vi "Vision Processing.vi"(2 "error in (no error)":errorcluster, 3 "Camera Type":enum16{"206", "1011"}(ring)=enum."1011", 4 "Camera Name":string="Camera") -> (0 "Target Info":T1(array[cluster]))   [LabVIEW 2012]
uses:
  Robot Global Data.vi
  <vilib>/vision/NI_Vision_Development_Module.lvlib
panel:
  in  "View Zoom":bool
  in  "Make Target Info":T1(array[cluster])
  in  "Don't use camera?":bool=TRUE
  out "zoomed binary":T2(plugin-control)
  in  "View":bool
  in  "Area Size Limit":i32=444
  in  "Particle Count Limit":i32=8
  in  "Score Limits":T3={"Rect Coverage"=76.0, "Aspect Ratio"=70.0, "X Edge Strength"=60.0, "Y Edge Strength"=40.0}
  in  "Processing":enum32{"Color", "Intensity", "Intensity Open"}(tab)
  in  "Luminance":i32=200
  in  "Saturation":i32=50
  in  "Hue":i32(knob)=121 scale=0.0..255.0
  in  "Margins":cluster{"Hue":i32, "Sat":i32, "Lum":i32}={"Hue"=40, "Sat"=40, "Lum"=20} {"Sat" scale=0.0..40.0; "Lum" scale=0.0..40.0; "Hue" scale=0.0..40.0}
  in  "Range":cluster{"Lower value":sgl, "Upper value":sgl}={"Lower value"=150.0, "Upper value"=255.0} {"Lower value" scale=0.0..255.0; "Upper value" scale=0.0..255.0}
  in  "Range":cluster{"Lower value":sgl, "Upper value":sgl}={"Lower value"=150.0, "Upper value"=255.0} {"Lower value" scale=0.0..255.0; "Upper value" scale=0.0..255.0}
  in  "View":bool
  out "Processed Image":T2(plugin-control)
  out "Original Image":T2(plugin-control)
  # "Instructions:\nProcessing the reflective tape that is illuminated by a ring light can be based\non color or light intensity.\nParticles within the image are scored by rectangle coverage, aspect ratio, and\nfor being hollow with a bold edge. A particle is considered a target if all scores\nare above the score limits. Particles can be annotated -- surrounded by\na rectangle and scores drawn to the left .\nTo control the number of particles being scored, use the count limit and the size\nlimit."
  # "To debug, Enable using the View button.\nFor color processing, you can click in the image to select the color for processing."
  # "Enable by clicking the View button.\nGreen scores are above the limit, orange are below. Inner/outer rect\nindicates all passed."
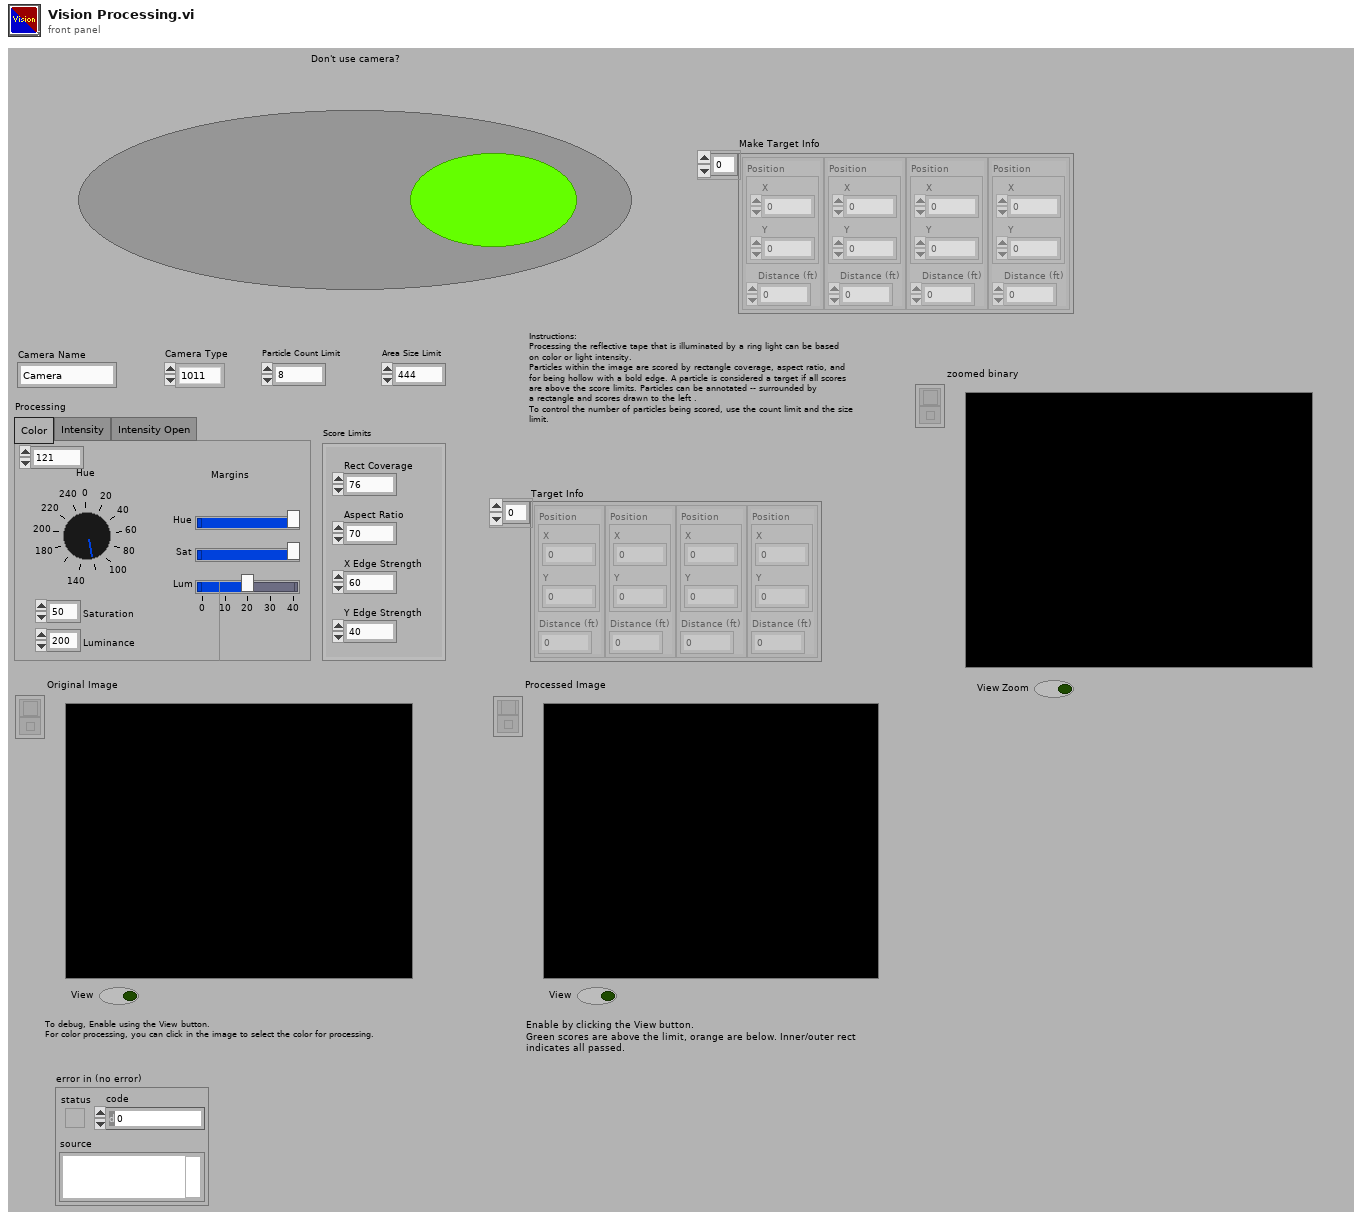
[diagram p1: front panel]
types:
  T1 = cluster{"Position":cluster{"X":dbl, "Y":dbl}, "Distance (ft)":dbl}[]
  T2 = typedef "IMAQ Image.ctl" = refnum<image>
  T3 = cluster{"Rect Coverage":dbl, "Aspect Ratio":dbl, "X Edge Strength":dbl, "Y Edge Strength":dbl}
  T4 = enum32{"AutoM", "Close", "Dilate", "Erode", "Gradient", "Gradient out", "Gradient in", "Hit miss", "Open", "PClose", "POpen", "Thick", "Thin"}
  T5 = typedef "Image Type" = u32
  T6 = typedef "WPI_CameraDevRef.ctl" = cluster{"Camera Address":string, "CameraStatus":errorcluster, "Acquire Image Notifier":refnum<notifier>}
  T7 = typedef "WPI_CameraImageSize.ctl" = enum16{"640x480", "320x240", "160x120"}
  T8 = cluster{cluster{"Left":dbl, "Top":dbl, "Right":dbl, "Bottom":dbl}, dbl[]}[]
  T9 = cluster{"Left":dbl, "Top":dbl, "Right":dbl, "Bottom":dbl}
  T10 = cluster{"Target Center (-1 to 1)":cluster{"X":dbl, "Y":dbl}, "Distance (ft)":dbl}
  T11 = cluster{"Target Center (-1 to 1)":cluster{"X":dbl, "Y":dbl}, "Distance (ft)":dbl}[]
  T12 = cluster{"Scored Particle Info[0]":cluster{cluster{"Left":dbl, "Top":dbl, "Right":dbl, "Bottom":dbl}, dbl[]}, "Scored Particle Info[1]":cluster{cluster{"Left":dbl, "Top":dbl, "Right":dbl, "Bottom":dbl}, dbl[]}, "Scored Particle Info[2]":cluster{cluster{"Left":dbl, "Top":dbl, "Right":dbl, "Bottom":dbl}, dbl[]}, "Scored Particle Info[3]":cluster{cluster{"Left":dbl, "Top":dbl, "Right":dbl, "Bottom":dbl}, dbl[]}, "Scored Particle Info[4]":cluster{cluster{"Left":dbl, "Top":dbl, "Right":dbl, "Bottom":dbl}, dbl[]}, "Scored Particle Info[5]":cluster{cluster{"Left":dbl, "Top":dbl, "Right":dbl, "Bottom":dbl}, dbl[]}, "Scored Particle Info[6]":cluster{cluster{"Left":dbl, "Top":dbl, "Right":dbl, "Bottom":dbl}, dbl[]}, "Scored Particle Info[7]":cluster{cluster{"Left":dbl, "Top":dbl, "Right":dbl, "Bottom":dbl}, dbl[]}, "Scored Particle Info[8]":cluster{cluster{"Left":dbl, "Top":dbl, "Right":dbl, "Bottom":dbl}, dbl[]}}
  T13 = cluster{cluster{"Left":dbl, "Top":dbl, "Right":dbl, "Bottom":dbl}, dbl[]}
  T14 = cluster{"Position":cluster{"X":dbl, "Y":dbl}, "Distance (ft)":dbl}
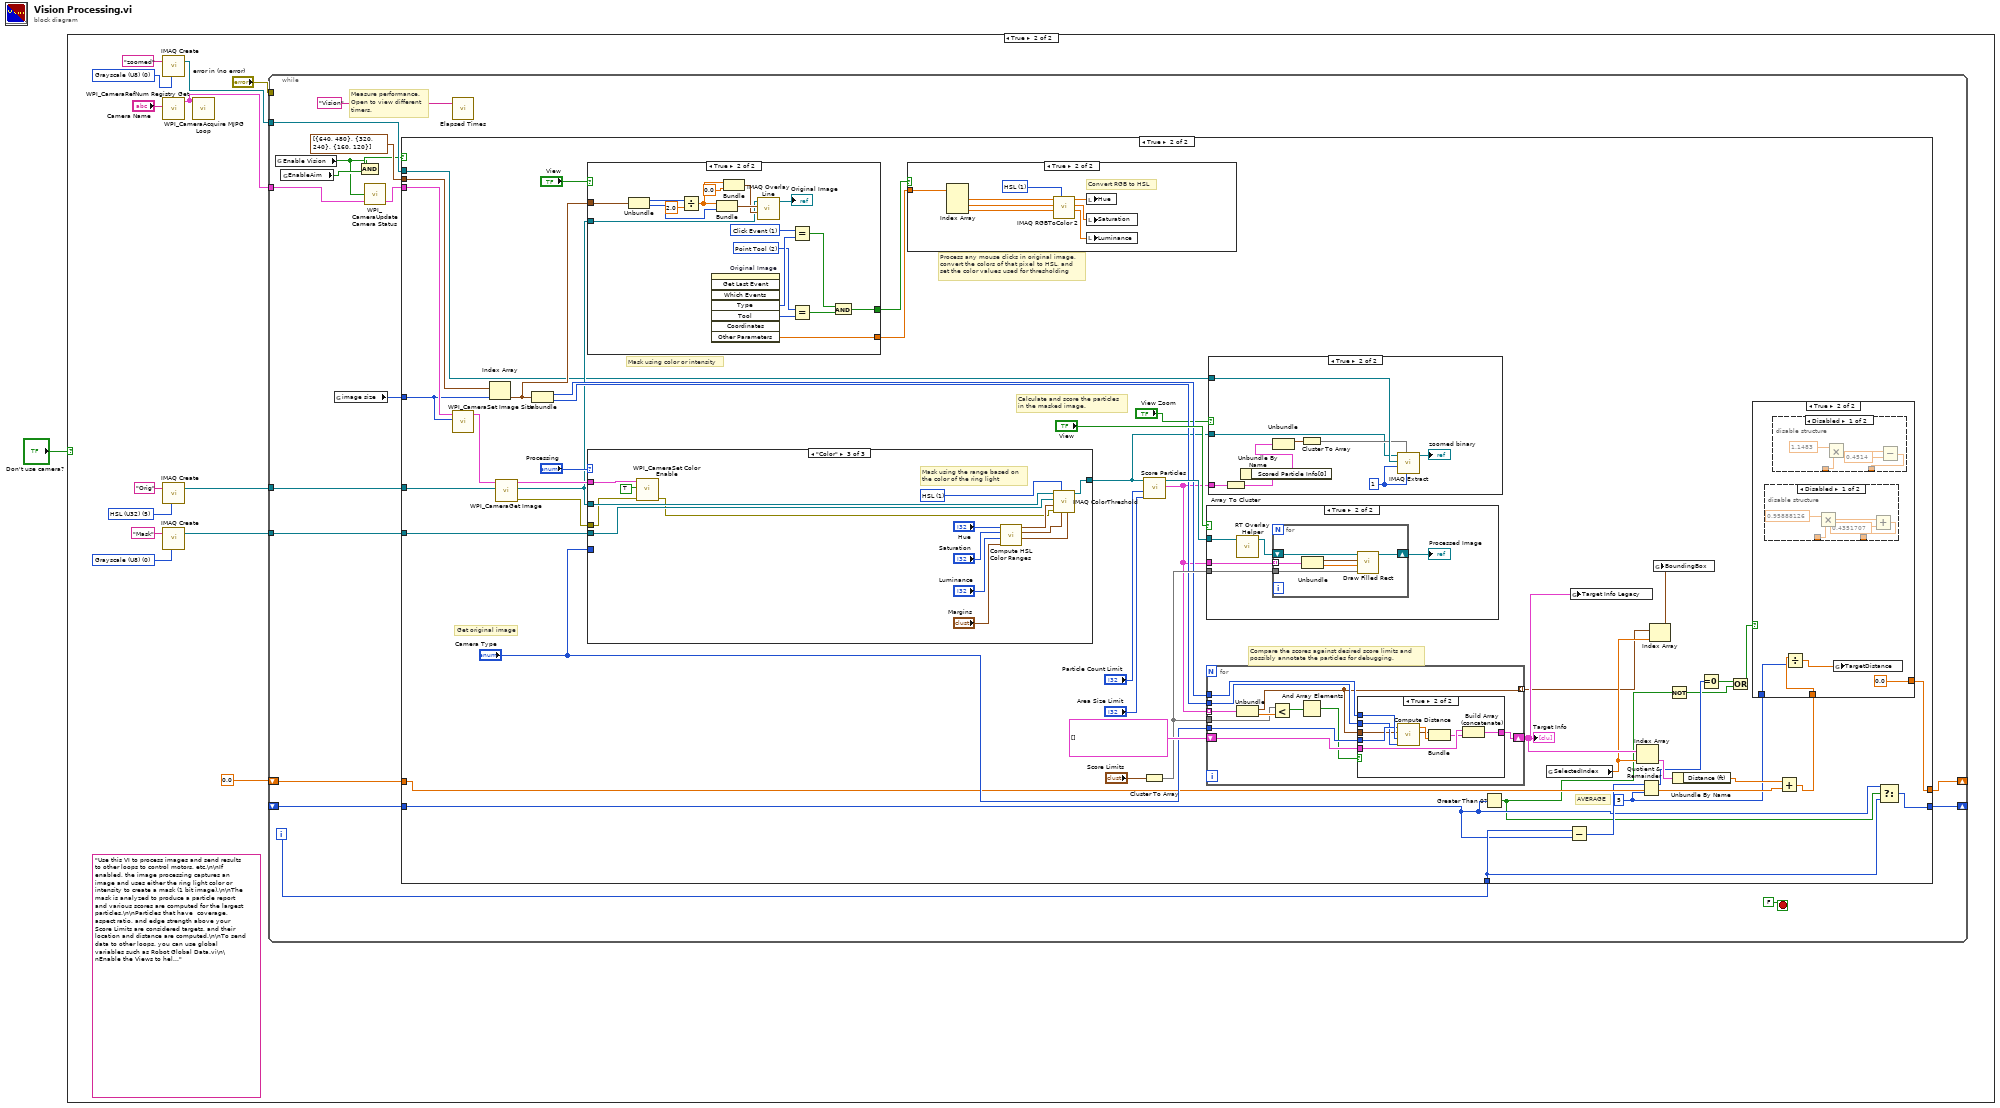
[diagram p0: block diagram]
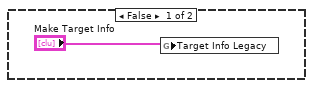
[diagram p2: hidden frame]
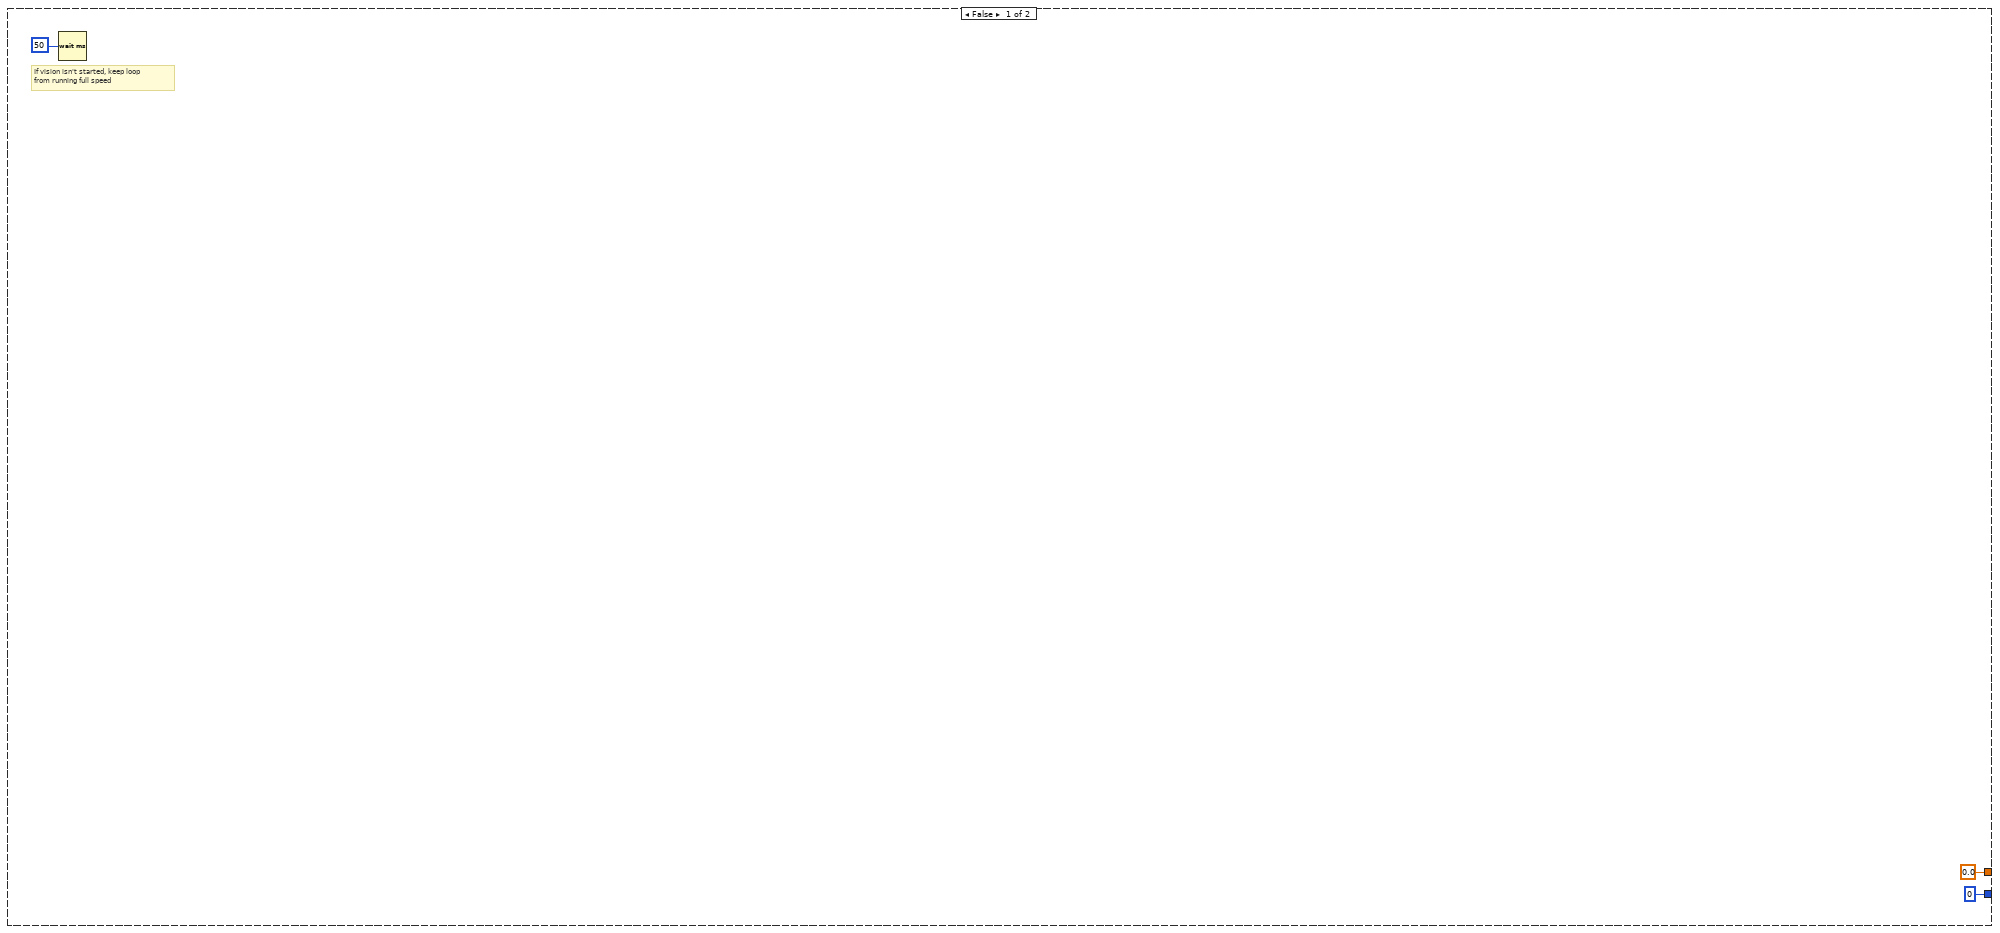
[diagram p3: hidden frame]
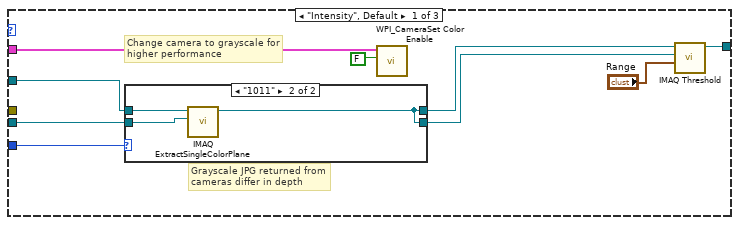
[diagram p9: hidden frame]
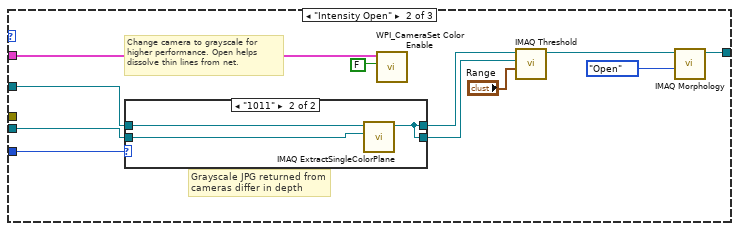
[diagram p11: hidden frame]
diagram:
  n1 = case shown="True" "Don't use camera?" {
    frame False {
      n2 = global write "Robot Global Data.vi" "Target Info Legacy"("Make Target Info") -> ()
    }
    frame True {
      w5 = T5 0 items=["Grayscale (U8)", "Grayscale (I16)", "Grayscale (SGL)", "Complex (CSG)", "RGB (U32)", "HSL (U32)", "RGB (U64)", "Grayscale (U16)"] ("Image Type")
      w9 = T5 0 items=["Grayscale (U8)", "Grayscale (I16)", "Grayscale (SGL)", "Complex (CSG)", "RGB (U32)", "HSL (U32)", "RGB (U64)", "Grayscale (U16)"] ("Image Type")
      (unwired) "Use this VI to process images and send results to other loops to control motors, etc.\n\nIf enabled, the image processing captures an image and uses either the ring light color or intensity to create a mask (1 bit image).\n\nThe mask is analyzed to produce a particle report and various scores are computed for the largest particles.\n\nParticles that have  coverage, aspect ratio, and edge strength above your Score Limits are considered targets, and their location and distance are computed.\n\nTo send data to other loops, you can use global variables such as Robot Global Data.vi\n\nEnable the Views to help debug color settings. Disable the View to speed up processing."
      w14 = T5 5 items=["Grayscale (U8)", "Grayscale (I16)", "Grayscale (SGL)", "Complex (CSG)", "RGB (U32)", "HSL (U32)", "RGB (U64)", "Grayscale (U16)"] ("Image Type")
      n3 = call "IMAQ Create"("Image Name"="zoomed", "Image Type"=w5) -> ("New Image"=w4:T2)  [unwired: 2 in, 2 out]
      n4 = call <vilib>:"WPI_CameraRefNum Registry Get.vi"("refnum name"="Camera Name") -> ("CameraDevRef"=w11:T6)  [unwired: 9 in, 1 out]
      n5 = call "IMAQ Create"("Image Name"="Orig", "Image Type"=w14) -> ("New Image"=w13:T2)  [unwired: 2 in, 2 out]
      n6 = call "IMAQ Create"("Image Name"="Mask", "Image Type"=w9) -> ("New Image"=w7:T2)  [unwired: 2 in, 2 out]
      n7 = call <vilib>:"WPI_CameraAcquire MJPG Loop.vi"("CameraDevRef"=w11) -> ()  [unwired: 11 in]
      n8 = while {
        tunnel: w13 -> [w31]
        tunnel: w11 -> [w30]
        tunnel: "error in (no error)" -> [_]
        tunnel: w7 -> [w26]
        tunnel: w4 -> [w24]
        shift-right: [w20] -> _
        shift-left: 0.0 -> [w21]
        shift-right: [w18] -> _
        shift-left: _ -> [w17]
        i -> [w19]
        stop <- FALSE stop-if-true
        # "Measure performance.\nOpen to view different\ntimers."
        n9 = global read "Robot Global Data.vi" "Enable Vision"() -> (w16:bool)
        n10 = global read "Robot Global Data.vi" "EnableAim"() -> (w23:bool)
        n11 = global read "Robot Global Data.vi" "image size"() -> (w27:T7)
        n12 = And(x=w16, y=w23) -> (x .and. y?=w22:bool)
        n13 = call <vilib>:"WPI_CameraUpdate Camera Status.vi"("CameraDevRef In"=w30, "Enable Vision"=w16) -> ("CameraDevRef Out"=w29:T6)  [unwired: 3 in]
        n14 = case shown="True" w22 {
          tunnel: w31 -> [_ w58]
          tunnel: w29 -> [_ w71]
          tunnel: w27 -> [_ w67]
          tunnel: w26 -> [_ w63]
          tunnel: cluster{i32, i32}[] [{640, 480}, {320, 240}, {160, 120}] -> [_ w66]
          tunnel: w24 -> [_ w59]
          tunnel: w21 -> [_ w52]
          tunnel: [0.0 w49] -> w20
          tunnel: w19 -> [_ w47]
          tunnel: [0 w46] -> w18
          tunnel: w17 -> [_ w42]
          frame False {
            # "If vision isn't started, keep loop\nfrom running full speed"
            n15 = Wait (ms)(milliseconds to wait=u32 50) -> ()  [unwired: 1 out]
          }
          frame True {
            w37 = 5 ("y")
            # "AVERAGE"
            # "Compare the scores against desired score limits and\npossibly annotate the particles for debugging."
            # "Process any mouse clicks in original image,\nconvert the colors of that pixel to HSL, and\nset the color values used for thresholding"
            # "Calculate and score the particles\nin the masked image."
            # "Mask using color or intensity"
            # "Get original image"
            n16 = call <vilib>:"WPI_CameraSet Image Size.vi"("Image Size"=w67, "CameraDevRef"=w71) -> ("CameraDevRef Out"=w72:T6)  [unwired: 8 in, 1 out]
            n17 = Index Array(array=w66, index=w67) -> (element=w60:cluster{i32, i32})
            n18 = call <vilib>:"WPI_CameraGet Image.vi"("Image"=w58, "CameraDevRef"=w72) -> ("error out"=w73:errorcluster, "Image Out"=w61:T2, "CameraDevRef Out"=w74:T6)  [unwired: 7 in]
            n19 = Unbundle(w60) -> (w65:i32, w64:i32)
            n20 = case shown="True" "View" {
              tunnel: w61 -> [_ w173]
              tunnel: [_ w184] -> w69
              tunnel: [_ w181] -> w68
              tunnel: w60 -> [_ w172]
              frame False {
              }
              frame True {
                w182 = 2 items=["None", "Selection Tool", "Point Tool", "Line Tool", "Rectangle Tool", "Oval Tool", "Polygon Tool", "ClosedFreehandTool", "Annulus Tool", "Rotated Rectangle Tool", "Zoom Tool", "Pan Tool", "Polyline Tool", "Freehand Tool"] ("Tool")
                w183 = 1 items=["No Event"=0, "Click Event"=1, "Draw Event"=2, "Size Event"=4, "Scroll Event"=5, "Double Click Event"=8] ("Type")
                n21 = Unbundle(w172) -> (w176:i32, w175:i32)
                n22 = Divide(x=w176, y=2.0) -> (x/y=w174:dbl)
                n23 = invoke on="Original Image" class="ImageControl" method="Get Last Event"() -> ("Type"=w185:i32, "Tool"=w188:i32, "Other Parameters"=w181:sgl[])  [unwired: 8 in, 5 out]
                n24 = Bundle(w174, w175) -> (w179:cluster{dbl, i32})  [unwired: 1 in]
                n25 = Bundle(w174, "element"=0.0) -> (w177:cluster{dbl, "element":dbl})  [unwired: 1 in]
                n26 = call "IMAQ Overlay Line"("End Point"=w177, "Start Point"=w179, "Image"=w173) -> ("Image Out"=→"Original Image":T2)  [unwired: 7 in, 1 out]
                n27 = Equal?(x=w183, y=w185) -> (x = y?=w186:bool)
                n28 = Equal?(x=w182, y=w188) -> (x = y?=w187:bool)
                n29 = And(x=w186, y=w187) -> (x .and. y?=w184:bool)
              }
            }
            n30 = case shown="\"Color\"" "Processing" {
              tunnel: w61 -> [w119 w131 w159]
              tunnel: [w122 w136 w158] -> w56
              tunnel: w74 -> [w120 w134 w149]
              tunnel: w73 -> [_ _ w146]
              tunnel: w63 -> [w118 w132 w147]
              tunnel: "Camera Type" -> [w117 w133 _]
              frame "Intensity", Default {
                # "Grayscale JPG returned from\ncameras differ in depth"
                # "Change camera to grayscale for\nhigher performance"
                n31 = case shown="\"1011\"" w117 {
                  tunnel: w119 -> [w125 w128]
                  tunnel: w118 -> [w124 w127]
                  tunnel: [w125 w126] -> w116
                  tunnel: [w124 w126] -> w115
                  frame "206", Default {
                  }
                  frame "1011" {
                    n32 = call "IMAQ ExtractSingleColorPlane"("Image Dst"=w127, "Image Src"=w128) -> ("Image Dst Out"=w126:T2)  [unwired: 8 in, 1 out]
                  }
                }
                n33 = call <vilib>:"WPI_CameraSet Color Enable.vi"("Color Enabled"=FALSE, "CameraDevRef"=w120) -> ()  [unwired: 8 in, 2 out]
                n34 = call "IMAQ Threshold"("Range"="Range", "Image Dst"=w115, "Image Src"=w116) -> ("Image Dst Out"=w122:T2)  [unwired: 3 in, 5 out]
              }
              frame "Intensity Open" {
                # "Grayscale JPG returned from\ncameras differ in depth"
                # "Change camera to grayscale for\nhigher performance. Open helps\ndissolve thin lines from net."
                n35 = case shown="\"1011\"" w133 {
                  tunnel: w131 -> [w141 w144]
                  tunnel: w132 -> [w140 w143]
                  tunnel: [w141 w142] -> w130
                  tunnel: [w140 w142] -> w129
                  frame "206", Default {
                  }
                  frame "1011" {
                    n36 = call "IMAQ ExtractSingleColorPlane"("Image Dst"=w143, "Image Src"=w144) -> ("Image Dst Out"=w142:T2)  [unwired: 8 in, 1 out]
                  }
                }
                n37 = call <vilib>:"WPI_CameraSet Color Enable.vi"("Color Enabled"=FALSE, "CameraDevRef"=w134) -> ()  [unwired: 8 in, 2 out]
                n38 = call "IMAQ Threshold"("Range"="Range", "Image Dst"=w129, "Image Src"=w130) -> ("Image Dst Out"=w137:T2)  [unwired: 3 in, 5 out]
                n39 = call "IMAQ Morphology"("Operation"=T4."Open", "Image Src"=w137) -> ("Image Dst Out"=w136:T2)  [unwired: 8 in, 1 out]
              }
              frame "Color" {
                w157 = u16 1 items=["RGB", "HSL", "HSV", "HSI"] ("Color Mode")
                # "Mask using the range based on\nthe color of the ring light"
                n40 = call <vilib>:"WPI_CameraSet Color Enable.vi"("error in (no error)"=w146, "Color Enabled"=TRUE, "CameraDevRef"=w149) -> ("error out"=w145:errorcluster)  [unwired: 7 in, 1 out]
                n41 = call "Compute HSL Color Ranges.vi"("Margins"="Margins", "Luminance"="Luminance", "Saturation"="Saturation", "Hue"="Hue") -> ("Lum Range"=w154:cluster{i32, i32}, "Sat Range"=w155:cluster{i32, i32}, "Hue Range"=w156:cluster{i32, i32})  [unwired: 5 in]
                n42 = call "IMAQ ColorThreshold"("Blue or Luma or Val or Inten Range"=w154, "Green or Sat Range"=w155, "Color Mode"=w157, "error in (no error)"=w145, "Red or Hue Range"=w156, "Image Dst"=w147, "Image Src"=w159) -> ("Image Dst Out"=w158:T2)  [unwired: 3 in, 1 out]
              }
            }
            n43 = case shown="True" w69 {
              tunnel: w68 -> [_ w114]
              frame False {
              }
              frame True {
                w113 = u16 1 items=["RGB", "HSL", "HSV", "HSI", "CIE L*a*b*", "CIE XYZ"] ("Color Mode")
                # "Convert RGB to HSL"
                n44 = Index Array(array=w114) -> (element #1=w112:sgl, element #2=w110:sgl, element #3=w108:sgl)  [unwired: 3 in]
                n45 = call "IMAQ RGBToColor 2"("Color Mode"=w113, "Blue value"=w108, "Green value"=w110, "Red value"=w112) -> ("Blue or Luma or Val or Inten or Z or b*value"=w107:dbl, "Green or Sat or Y or a* value"=w109:dbl, "Red or Hue or X or L* value"=w111:dbl)  [unwired: 4 in, 1 out]
                n46 = local write "Hue"(w111) -> ()
                n47 = local write "Saturation"(w109) -> ()
                n48 = local write "Luminance"(w107) -> ()
              }
            }
            n49 = Cluster To Array(cluster="Score Limits") -> (array=w77:dbl[])
            n50 = call "Score Particles.vi"("Area Size Limit"="Area Size Limit", "Particle Count Limit"="Particle Count Limit", "Image Refnum in"=w56) -> ("Scored Particle Info"=w57:T8, "Image Refnum out"=w81:T2)  [unwired: 7 in]
            n51 = case shown="True" "View" {
              tunnel: w81 -> [_ w161]
              tunnel: w57 -> [_ w163]
              tunnel: w77 -> [_ w162]
              frame False {
              }
              frame True {
                n52 = call "RT Overlay Helper.vi"("Refnum in"=w161) -> ("Refnum out"=w164:T2)  [unwired: 10 in]
                n53 = for {
                  shift-right: [w169] -> w160
                  shift-left: w164 -> [w170]
                  tunnel: w163 -> [w166] mode=indexing
                  tunnel: w162 -> [w165]
                  n54 = Unbundle(w166) -> (w167:T9, w168:dbl[])
                  n55 = call "Draw Filled Rect.vi"("Limits"=w165, "Scores"=w168, "Bounding Box"=w167, "image in"=w170) -> ("image out"=w169:T2)  [unwired: 7 in]
                }
                "Processed Image" <- w160
              }
            }
            n56 = for {
              shift-right: [w198] -> w55
              shift-left: T1 [] -> [w199]
              tunnel: w65 -> [w197]
              tunnel: w57 -> [w196] mode=indexing
              tunnel: w77 -> [w191]
              tunnel: "Camera Type" -> [w195]
              tunnel: w64 -> [w190]
              tunnel: [w189] -> w44 mode=indexing
              n57 = Unbundle(w196) -> (w189:T9, w192:dbl[])
              n58 = Less?(x=w191, y=w192) -> (x < y?=w194:bool[])
              n59 = And Array Elements(Boolean array=w194) -> (logical AND=w193:bool)
              n60 = case shown="True" w193 {
                tunnel: w199 -> [w200 w209]
                tunnel: [w200 w208] -> w198
                tunnel: w189 -> [_ w201]
                tunnel: w197 -> [_ w206]
                tunnel: w195 -> [_ w204]
                tunnel: w190 -> [_ w203]
                frame False {
                }
                frame True {
                  n61 = call "Compute Distance.vi"("Y Image Resolution"=w203, "X Image Resolution"=w206, "Bounding Box"=w201, "Camera Type"=w204) -> ("Target Center (-1 to 1)"=w202:cluster{"X":dbl, "Y":dbl}, "Distance (ft)"=w205:dbl)  [unwired: 6 in]
                  n62 = Bundle("Target Center (-1 to 1)"=w202, "Distance (ft)"=w205) -> (w207:T10)  [unwired: 1 in]
                  n63 = Build Array (concatenate)(w209, w207) -> (w208:T11)
                }
              }
            }
            "Target Info" <- w55
            n64 = case shown="True" "View Zoom" {
              tunnel: w59 -> [_ w91]
              tunnel: w57 -> [_ w90]
              tunnel: w56 -> [_ w87]
              frame False {
              }
              frame True {
                w85 = 1 ("X Step Size")
                n65 = Array To Cluster(array=w90) -> (cluster=w84:T12)
                n66 = Unbundle By Name(w84) -> ("Scored Particle Info[0]"=w83:T13)
                n67 = Unbundle(w83) -> (w89:T9)  [unwired: 1 out]
                n68 = Cluster To Array(cluster=w89) -> (array=w88:dbl[])
                n69 = call "IMAQ Extract"("Y Step Size"=w85, "Optional Rectangle"=w88, "X Step Size"=w85, "Image Dst"=w91, "Image Src"=w87) -> ("Image Dst Out"=→"zoomed binary":T2)  [unwired: 5 in, 1 out]
              }
            }
            n70 = Greater Than 0?(x=w42) -> (x > 0?=w39:bool)
            n71 = global read "Robot Global Data.vi" "SelectedIndex"() -> (w45:dbl)
            n72 = Subtract(x=w47, y=w42) -> (x-y=w48:i32)
            n73 = global write "Robot Global Data.vi" "Target Info Legacy"(w55) -> ()
            n74 = Index Array(array=w55, index=w45) -> (element=w54:T14)
            n75 = Quotient & Remainder(x=w48, y=w37) -> (x-y*floor(x/y)=w41:i32)  [unwired: 1 out]
            n76 = Index Array(array=w44, index=w45) -> (element=w43:T9)
            n77 = global write "Robot Global Data.vi" "BoundingBox"(w43) -> ()
            n78 = Not(x=w39) -> (.not. x?=w38:bool)
            n79 = Unbundle By Name(w54) -> ("Distance (ft)"=w53:dbl)
            n80 = Equal To 0?(x=w41) -> (x = 0?=w50:bool)
            n81 = Or(x=w50, y=w38) -> (x .or. y?=w40:bool)
            n82 = Add(x=w53, y=w52) -> (x+y=w51:dbl)
            n83 = case shown="True" w40 {
              tunnel: w51 -> [w92 w96]
              tunnel: [w92 0.0] -> w49
              tunnel: w37 -> [_ w93]
              frame False {
              }
              frame True {
                n84 = disable-structure shown="Disabled" {
                  disable-tunnel: [w100 _] -> _
                  disable-tunnel: _ -> [w97 _]
                  frame Disabled {
                    n85 = Multiply(x=0.95888126, y=w97) -> (x*y=w101:dbl)
                    n86 = Add(x=w101, y=0.4351707) -> (x+y=w100:dbl)
                  }
                  frame Enabled {
                  }
                }
                n87 = disable-structure shown="Disabled" {
                  disable-tunnel: [w105 _] -> _
                  disable-tunnel: _ -> [w102 _]
                  frame Disabled {
                    n88 = Multiply(x=1.1483, y=w102) -> (x*y=w106:dbl)
                    n89 = Subtract(x=w106, y=0.4514) -> (x-y=w105:dbl)
                  }
                  frame Enabled {
                  }
                }
                n90 = Divide(x=w96, y=w93) -> (x/y=w94:dbl)
                n91 = global write "Robot Global Data.vi" "TargetDistance"(w94) -> ()
              }
            }
            n92 = Select(t=w42, s=w39, f=w47) -> (s? t:f=w46:i32)
          }
        }
        n93 = call "Elapsed Times.vi"("Call Name"="Vision") -> ()  [unwired: 2 in, 1 out]
      }
    }
  }
